vi "Read Saving data.vi"(8 "error in (no error)":errorcluster, 11 "Abstract Saver in":refnum<class "Abstract Saver.lvclass">) -> (0 "error out":errorcluster, 2 "Saving data":bool, 3 "Abstract Saver out":refnum<class "Abstract Saver.lvclass">)   [LabVIEW 2016, in "Data Saving.lvlib" / "Abstract Saver.lvclass"]
uses:
  Abstract Saver.lvclass
  Abstract Saver.lvclass/Abstract Saver.ctl
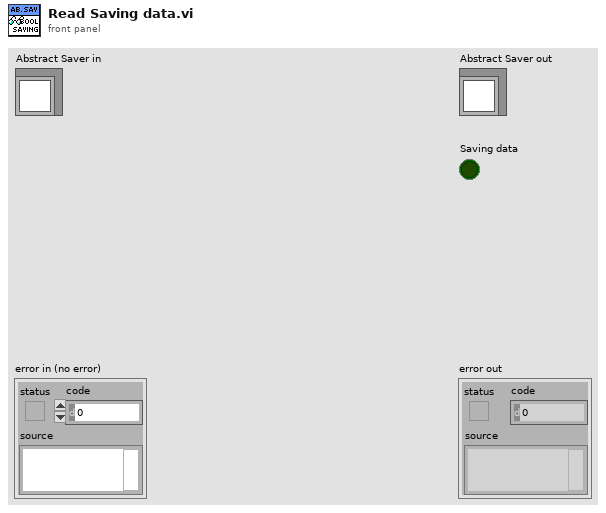
[diagram p1: front panel]
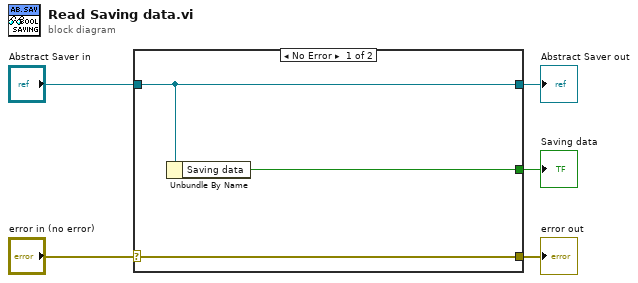
[diagram p0: block diagram]
diagram:
  n1 = case shown="No Error" "error in (no error)" {
    selector: "error in (no error)" -> [w8 w9]
    tunnel: [w8 w9] -> w4
    tunnel: [w7 w10] -> w2
    tunnel: "Abstract Saver in" -> [w7 w10]
    tunnel: [w6 _] -> w1
    frame No Error {
      n2 = Unbundle By Name(w7) -> ("Saving data"=w6:bool)
    }
    frame Error {
    }
  }
  "error out" <- w4
  "Abstract Saver out" <- w2
  "Saving data" <- w1
